vi "Lidar Encoder Counter.vi"   [LabVIEW 2009]
uses:
  Motor Control Global.vi
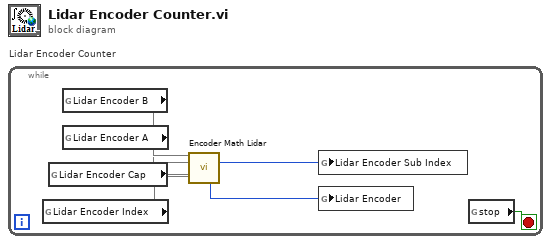
[diagram p0: block diagram]
diagram:
  n1 = while "Lidar Encoder Counter" {
    stop <- w7 stop-if-true
    n2 = global read "Motor Control Global.vi" "Lidar Encoder Index"() -> (w4)
    n3 = global read "Motor Control Global.vi" "Lidar Encoder Cap"() -> (w1)
    n4 = global read "Motor Control Global.vi" "Lidar Encoder B"() -> (w6)
    n5 = global read "Motor Control Global.vi" "Lidar Encoder A"() -> (w5)
    n6 = call "Encoder Math Lidar.vi"("Encoder B"=w6, "Encoder A"=w5, "Index Point"=w1, "Encoder Index"=w4) -> ("Count Zeroed at Index"=w2:i32, "Current count"=w3:i32)  [unwired: 8 in, 2 out]
    n7 = global write "Motor Control Global.vi" "Lidar Encoder Sub Index"(w2) -> ()
    n8 = global write "Motor Control Global.vi" "Lidar Encoder"(w3) -> ()
    n9 = global read "Motor Control Global.vi" "stop"() -> (w7:bool)
  }
